vi "Read Output Channels[].vi"(8 "error in (no error)":errorcluster, 11 "Plugin_UI in":refnum<class "Plugin_UI.lvclass">) -> (0 "error out":errorcluster, 2 "Output Channels[]":refnum<class "Output Channels.lvclass">[](array[class]), 3 "Plugin_UI out":refnum<class "Plugin_UI.lvclass">)   [LabVIEW 2020, in "Plugin.lvlib" / "Plugin_UI.lvclass"]
doc: "Read output channels."
uses:
  Plugin_UI.lvclass
  Channels/Output Channels/Output Channels.lvclass
  Plugin_UI.lvclass/Plugin_UI.ctl
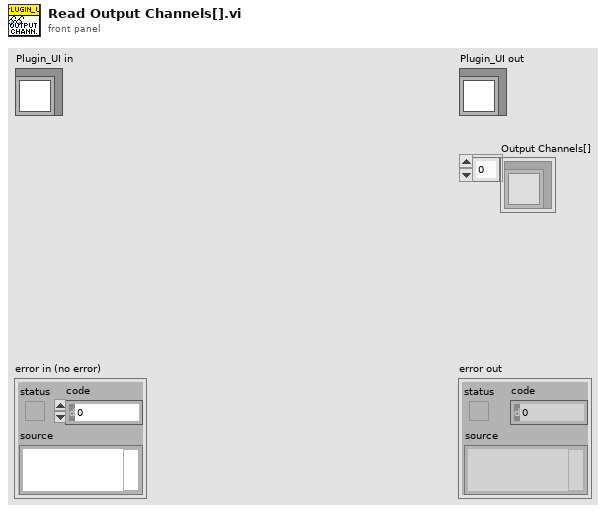
[diagram p1: front panel]
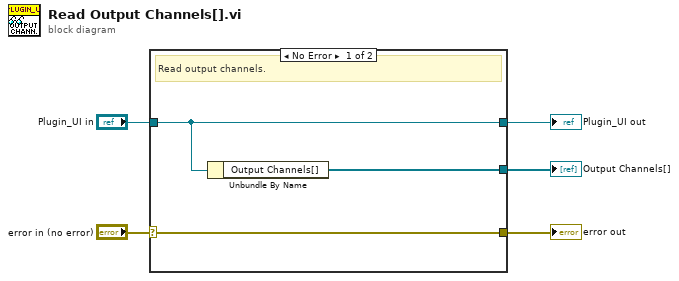
[diagram p0: block diagram]
diagram:
  n1 = case shown="No Error" "error in (no error)" {
    selector: "error in (no error)" -> [w8 w9]
    tunnel: [w8 w9] -> w4
    tunnel: [w7 w10] -> w2
    tunnel: "Plugin_UI in" -> [w7 w10]
    tunnel: [w6 _] -> w1
    frame No Error {
      # "Read output channels."
      n2 = Unbundle By Name(w7) -> ("Output Channels[]"=w6:refnum<class "Output Channels.lvclass">[])
    }
    frame Error {
    }
  }
  "error out" <- w4
  "Plugin_UI out" <- w2
  "Output Channels[]" <- w1
